vi "fd bitrate c2s.vi"(1 "cluster":T1) -> (0 "string":string)   [LabVIEW 2024, in "atsj peakcan basic.lvlib"]
uses:
  atsj peakcan basic.lvlib
  fd bitrate.ctl
  clock frequency.ctl
  fd bitrate parameters.ctl
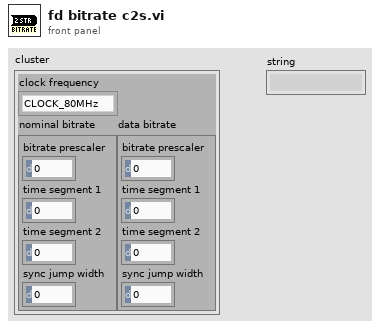
[diagram p1: front panel]
types:
  T1 = typedef "atsj peakcan basic.lvlib/fd bitrate.ctl" = cluster{"clock frequency":T2, "nominal bitrate":T3, "data bitrate":T3}
  T2 = typedef "atsj peakcan basic.lvlib/clock frequency.ctl" = enum16{"CLOCK_80MHz", "CLOCK_60MHz", "CLOCK_40MHz", "CLOCK_30MHz", "CLOCK_24MHz", "CLOCK_20MHz"}
  T3 = typedef "atsj peakcan basic.lvlib/fd bitrate parameters.ctl" = cluster{"bitrate prescaler":u16, "time segment 1":u16, "time segment 2":u16, "sync jump width":u16}
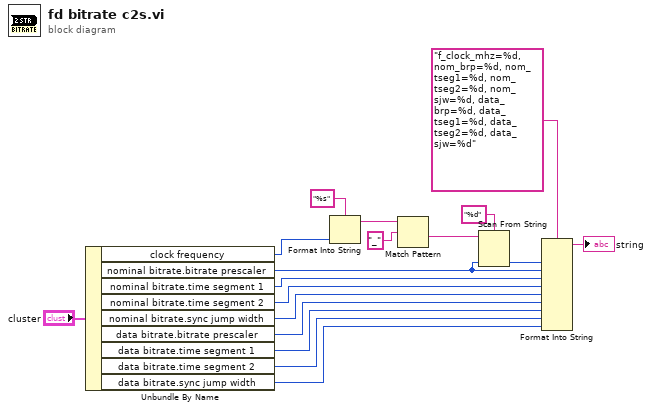
[diagram p0: block diagram]
diagram:
  n1 = Unbundle By Name("cluster") -> ("clock frequency"=w16:T2, "nominal bitrate.bitrate prescaler"=w1:u16, "nominal bitrate.time segment 1"=w9:u16, "nominal bitrate.time segment 2"=w8:u16, "nominal bitrate.sync jump width"=w7:u16, "data bitrate.bitrate prescaler"=w6:u16, "data bitrate.time segment 1"=w5:u16, "data bitrate.time segment 2"=w4:u16, "data bitrate.sync jump width"=w3:u16)
  n2 = Format Into String(format string="%s", w16) -> (resulting string=w14:string)  [unwired: 2 in, 1 out]
  n3 = Match Pattern(string=w14, regular expression="_") -> (after substring=w12:string)  [unwired: 1 in, 3 out]
  n4 = Scan From String(format string="%d", input string=w12, default 1=w1) -> (output 1=w10:u16)  [unwired: 2 in, 3 out]
  n5 = Format Into String(format string="f_clock_mhz=%d, nom_brp=%d, nom_tseg1=%d, nom_tseg2=%d, nom_sjw=%d, data_brp=%d, data_tseg1=%d, data_tseg2=%d, data_sjw=%d", w10, w1, w9, w8, w7, w6, w5, w4, w3) -> (resulting string=→"string":string)  [unwired: 2 in, 1 out]
